vi "WriteModuleToFile (SubVI).vi"(0 "Module ID":string="Test", 1 "Mark used for tracking":string="MarkC", 2 "Assembly step":string="Placement", 3 "User notes":string="Type your note here....", 4 "Current corner":string="CornerA", 5 "Fiducial Mark Position":dbl[](array[numeric])=[0.0, 0.0, 0.0], 6 "Temperature":dbl, 7 "error in (no error)":errorcluster, 8 "Module reports file path":path, 10 "Write to file":bool=TRUE) -> (13 "error out":errorcluster)   [LabVIEW 2016]
uses:
  <vilib>/Utility/config.llb/Write Key (String).vi
  <vilib>/Utility/config.llb/Write Key (Double).vi
  <vilib>/Utility/config.llb/NI_LVConfig.lvlib
panel:
  # "Module position information"
  # "General"
  # "(Date and time recorded)"
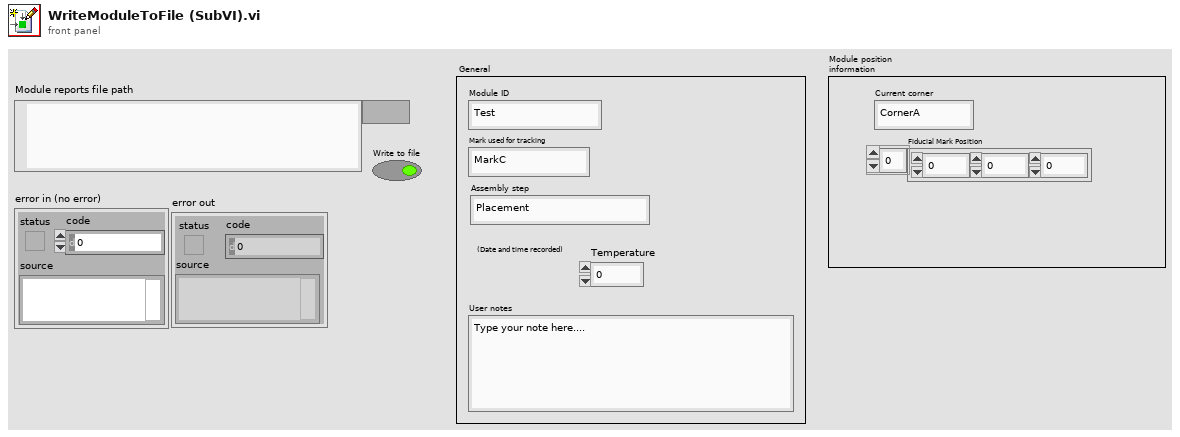
[diagram p1: front panel]
types:
  T1 = typedef "NI_LVConfig.lvlib/Config Data RefNum.ctl" = refnum<k1>
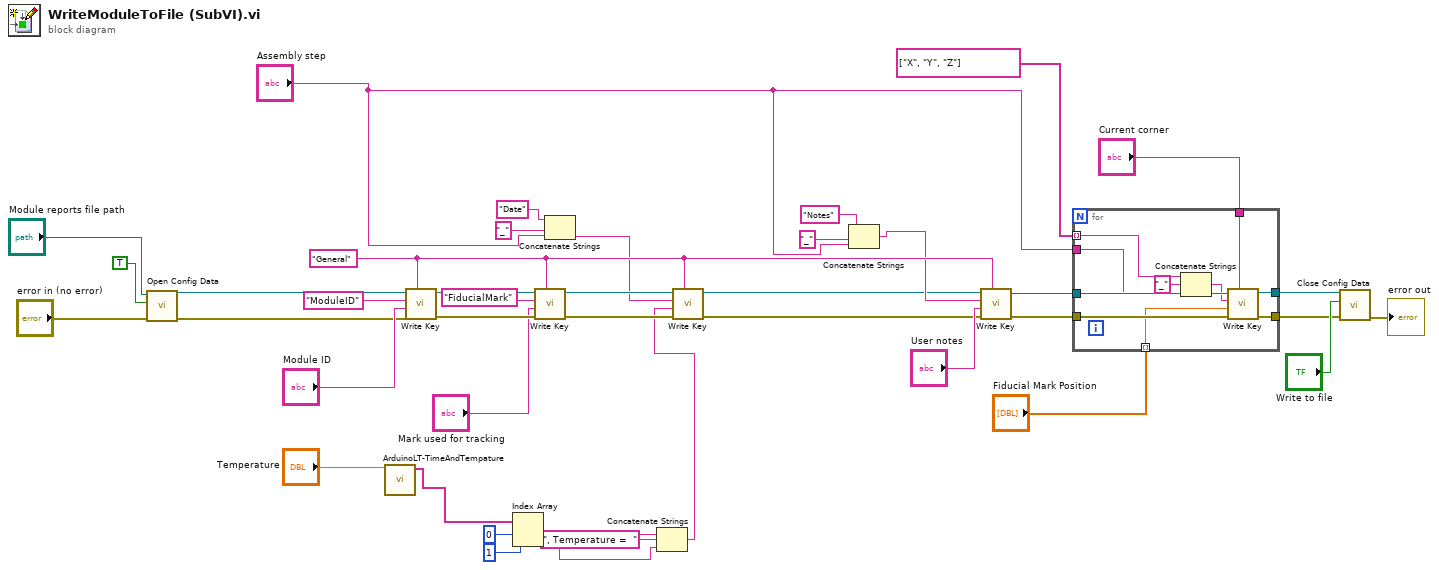
[diagram p0: block diagram]
diagram:
  w26 = "General" ("section")
  n1 = call <vilib>:"Open Config Data.vi"("error in (no error)"="error in (no error)", "create file if necessary (T)"=TRUE, "configuration file path"="Module reports file path") -> ("error out"=w35:errorcluster, "refnum"=w38:T1)  [unwired: 6 in, 1 out]
  n2 = call "ArduinoLT-TimeAndTempature.vi"("Temperature"="Temperature") -> ("str( Time, Temp )"=w7:string[])  [unwired: 8 in, 2 out]
  n3 = call-poly <vilib>:"Write Key.vi"("section"=w26, "error in (no error)"=w35, "value"="Module ID", "key"="ModuleID", "refnum"=w38) -> ("error out"=w32:errorcluster, "refnum out"=w34:T1)  [unwired: 4 in, 1 out]
  n4 = Index Array(array=w7, index #1=0 ("index"), index #2=1 ("index")) -> (element #1=w4:string, element #2=w3:string)
  n5 = call-poly <vilib>:"Write Key.vi"("section"=w26, "error in (no error)"=w32, "value"="Mark used for tracking", "key"="FiducialMark", "refnum"=w34) -> ("error out"=w25:errorcluster, "refnum out"=w27:T1)  [unwired: 4 in, 1 out]
  n6 = Concatenate Strings("Date" ("key"), "_" ("string"), "Assembly step") -> (w15:string)
  n7 = Concatenate Strings(w4, ", Temperature =  " ("string"), w3) -> (w1:string)
  n8 = call-poly <vilib>:"Write Key.vi"("section"=w26, "error in (no error)"=w25, "value"=w1, "key"=w15, "refnum"=w27) -> ("error out"=w8:errorcluster, "refnum out"=w9:T1)  [unwired: 4 in, 1 out]
  n9 = Concatenate Strings("Notes" ("key"), "_" ("string"), "Assembly step") -> (w10:string)
  n10 = call-poly <vilib>:"Write Key.vi"("section"=w26, "error in (no error)"=w8, "value"="User notes", "key"=w10, "refnum"=w9) -> ("error out"=w31:errorcluster, "refnum out"=w30:T1)  [unwired: 4 in, 1 out]
  n11 = for {
    tunnel: w31 -> [w51]
    tunnel: w30 -> [w50]
    tunnel: "Fiducial Mark Position" -> [w48] mode=indexing
    tunnel: string[] ["X", "Y", "Z"] -> [w46] mode=indexing
    tunnel: [w45] -> w21
    tunnel: [w44] -> w22
    tunnel: "Assembly step" -> [w43]
    tunnel: "Current corner" -> [w42]
    n12 = Concatenate Strings(w46, "_" ("string"), w43) -> (w49:string)
    n13 = call-poly <vilib>:"Write Key.vi"("section"=w42, "error in (no error)"=w51, "value"=w48, "key"=w49, "refnum"=w50) -> ("error out"=w45:errorcluster, "refnum out"=w44:T1)  [unwired: 4 in, 1 out]
  }
  n14 = call <vilib>:"Close Config Data.vi"("error in (no error)"=w21, "write file if changed (T)"="Write to file", "refnum"=w22) -> ("error out"=→"error out":errorcluster)  [unwired: 7 in, 1 out]
